vi "sv_Compute Weighting Relative Response (Octave).vi"(0 "octave spectrum":T1, 7 "weighting filter":u16(ring) items=["Linear", "A-weighting", "B-weighting", "C-weighting", "ITU-R 468-4", "Dolby", "CCITT", "C-message"], 9 "octave info in":T2={"standard"=enum."ANSI S1.11", "bandwidth"=enum."1 octave", "low band"=0, "high band"=0, "weighting filter"=0, "dB reference"=0.0, "dB On"=FALSE, "unit label"="", "channel name"="", "description"="", "engineering units"=1, "custom label"="", "spectrum type"=enum."magnitude", "spectral density"=FALSE, "filters settled"=FALSE} {"engineering units" items=["custom..."=0, "V"=1, "A"=21, "C"=30, "pC"=31, "s"=32, "-"=29, "Pa"=2, "N"=20, "g"=3, "m/s^2"=4, "m/s"=5, "m"=6, "mm/s"=12, "mm"=13, "micron/s"=14, "micron"=15, "in/s^2"=7, "in/s"=8, "in"=9, "mil/s"=10, "mil"=11, "rad/s^2"=16, "rad/s"=17, "rad"=18, "deg/s^2"=26, "deg/s"=27, "deg"=28, "RPM"=22, "cycle/s^2"=23, "Hz"=24, "cycle"=25, "strain"=19]; "dB reference" format="%.2e"; "weighting filter" items=["Linear", "A-weighting", "B-weighting", "C-weighting", "ITU-R 468-4", "Dolby", "CCITT", "C-message", "Wb", "Wc", "Wd", "We", "Wf", "Wh", "Wj", "Wk", "Wm", "AES17 20 kHz lowpass", "AES17 40 kHz lowpass", "AES17 20 kHz highpass", "AES17 40 kHz highpass"]}, 11 "error in (no error)":errorcluster, 12 "reset":bool) -> (4 "weighted octave spectrum":T1, 10 "octave info out":T2={"standard"=enum."ANSI S1.11", "bandwidth"=enum."1 octave", "low band"=0, "high band"=0, "weighting filter"=0, "dB reference"=0.0, "dB On"=FALSE, "unit label"="", "channel name"="", "description"="", "engineering units"=1, "custom label"="", "spectrum type"=enum."magnitude", "spectral density"=FALSE, "filters settled"=FALSE} {"engineering units" items=["custom..."=0, "V"=1, "A"=21, "C"=30, "pC"=31, "s"=32, "-"=29, "Pa"=2, "N"=20, "g"=3, "m/s^2"=4, "m/s"=5, "m"=6, "mm/s"=12, "mm"=13, "micron/s"=14, "micron"=15, "in/s^2"=7, "in/s"=8, "in"=9, "mil/s"=10, "mil"=11, "rad/s^2"=16, "rad/s"=17, "rad"=18, "deg/s^2"=26, "deg/s"=27, "deg"=28, "RPM"=22, "cycle/s^2"=23, "Hz"=24, "cycle"=25, "strain"=19]; "dB reference" format="%.2e"; "weighting filter" items=["Linear", "A-weighting", "B-weighting", "C-weighting", "ITU-R 468-4", "Dolby", "CCITT", "C-message", "Wb", "Wc", "Wd", "We", "Wf", "Wh", "Wj", "Wk", "Wm", "AES17 20 kHz lowpass", "AES17 40 kHz lowpass", "AES17 20 kHz highpass", "AES17 40 kHz highpass"]}, 15 "error out":errorcluster)   [LabVIEW 2017]
uses:
  <vilib>/addons/_NISVFA/_Shared subVIs/Controls/svc_Octave Info.ctl
  <vilib>/addons/_NISVFA/_Shared subVIs/Controls/svc_Octave Standard.ctl
  <vilib>/addons/_NISVFA/_Shared subVIs/Controls/svc_Weighting Filter Text Ring.ctl
  <vilib>/addons/_NISVFA/_Shared subVIs/Controls/svc_Engineering Units Text Ring.ctl
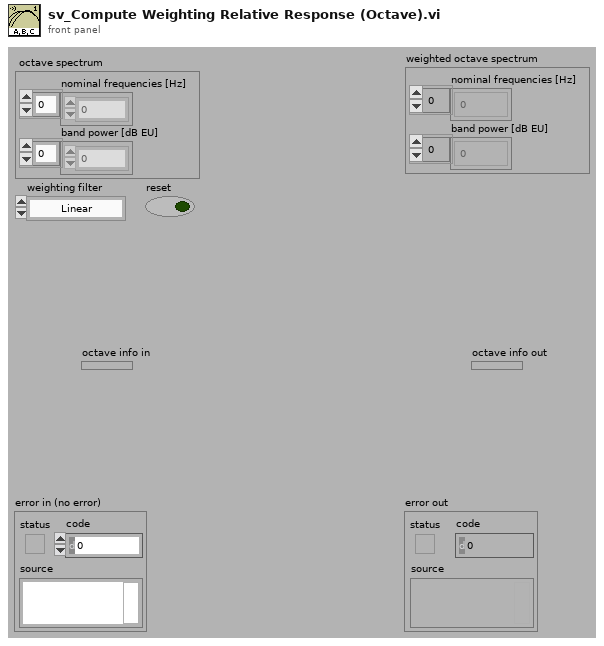
[diagram p1: front panel]
types:
  T1 = cluster{"nominal frequencies [Hz]":dbl[], "band power [dB EU]":dbl[]}
  T2 = typedef "svc_Octave Info.ctl" = cluster{"standard":T3, "bandwidth":enum16{"1 octave", "1/3 octave", "1/6 octave", "1/12 octave", "1/24 octave"}, "low band":i32, "high band":i32, "weighting filter":T4, "dB reference":dbl, "dB On":bool, "unit label":string, "channel name":string, "description":string, "engineering units":T5, "custom label":string, "spectrum type":enum16{"power", "magnitude"}, "spectral density":bool, "filters settled":bool}
  T3 = typedef "svc_Octave Standard.ctl" = enum16{"ANSI S1.11", "IEC 61260"}
  T4 = typedef "svc_Weighting Filter Text Ring.ctl" = u16
  T5 = typedef "svc_Engineering Units Text Ring.ctl" = u16
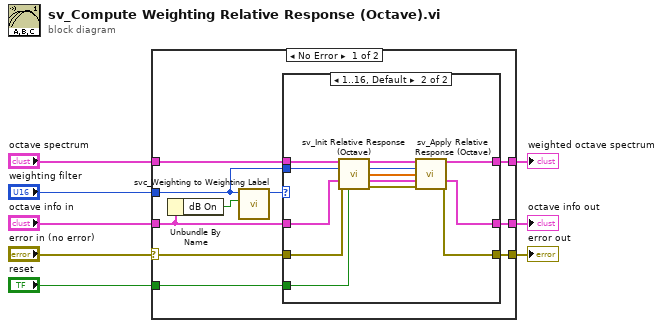
[diagram p0: block diagram]
diagram:
  n1 = case shown="No Error" "error in (no error)" {
    selector: "error in (no error)" -> [w11 w35]
    tunnel: "reset" -> [w18 _]
    tunnel: "weighting filter" -> [w17 _]
    tunnel: "octave info in" -> [w10 w36]
    tunnel: "octave spectrum" -> [w16 w37]
    tunnel: [w14 w36] -> w4
    tunnel: [w13 w35] -> w3
    tunnel: [w12 w37] -> w2
    frame No Error {
      n2 = Unbundle By Name(w10) -> ("dB On"=w9:bool)
      n3 = call <vilib>:"svc_Weighting to Weighting Label.vi"("dB On (T)"=w9, "weighting filter"=w17) -> ("weighting enum"=w15:T4)  [unwired: 8 in, 1 out]
      n4 = case shown="1..16, Default" w15 {
        tunnel: [w21 w34] -> w12
        tunnel: w16 -> [w21 w33]
        tunnel: w11 -> [w20 w27]
        tunnel: [w20 w26] -> w13
        tunnel: w10 -> [w19 w28]
        tunnel: [w19 w22] -> w14
        tunnel: w17 -> [_ w25]
        tunnel: w18 -> [_ w29]
        frame 0 {
          # "Skip weighting if \nweighting == Linear"
        }
        frame 1..16, Default {
          n5 = call <vilib>:"sv_Init Relative Response (Octave).vi"("octave spectrum"=w33, "weighting filter"=w25, "octave info"=w28, "error in (no error)"=w27, "reset"=w29) -> ("dup octave spectrum"=w32:T1, "dup weighting filter"=w24:u16, "relative response"=w23:dbl[], "dup octave info"=w30:T2, "error out"=w31:errorcluster)  [unwired: 6 in]
          n6 = call <vilib>:"sv_Apply Relative Response (Octave).vi"("octave spectrum"=w32, "weighting filter"=w24, "relative response"=w23, "octave info in"=w30, "error in (no error)"=w31) -> ("weighted octave spectrum"=w34:T1, "octave info out"=w22:T2, "error out"=w26:errorcluster)  [unwired: 8 in]
        }
      }
    }
    frame Error {
    }
  }
  "octave info out" <- w4
  "error out" <- w3
  "weighted octave spectrum" <- w2
